vi "EJERCICIO 2 DE LOGICA COMBINACIONAL.vi"() -> ()   [LabVIEW 2013]
panel:
  out "Boolean":bool
  in  "C":bool
  in  "B":bool
  in  "A":bool
  # "universidad de cundinamarca\ningenieria de sistemas \nandy leandro camargo \nelectiva pro IV"
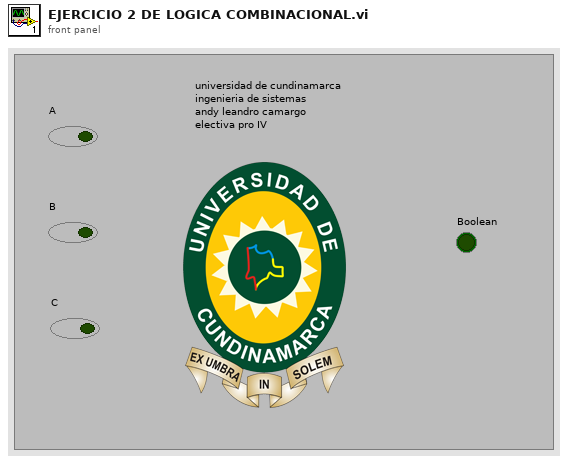
[diagram p1: front panel]
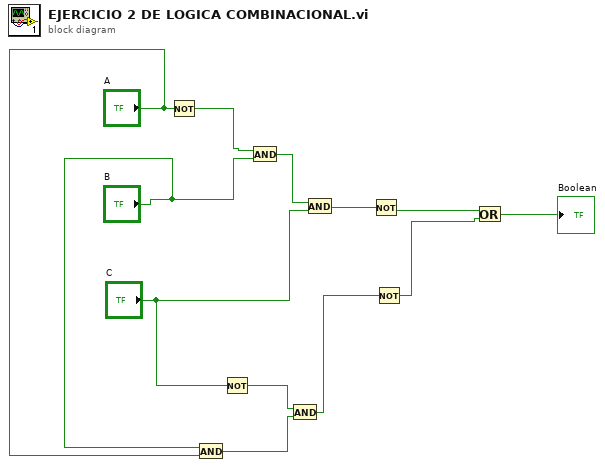
[diagram p0: block diagram]
diagram:
  n1 = Not(x="A") -> (.not. x?=w12:bool)
  n2 = And(x="B", y="A") -> (x .and. y?=w2:bool)
  n3 = Not(x="C") -> (.not. x?=w3:bool)
  n4 = And(x=w12, y="B") -> (x .and. y?=w11:bool)
  n5 = And(x=w3, y=w2) -> (x .and. y?=w1:bool)
  n6 = And(x=w11, y="C") -> (x .and. y?=w8:bool)
  n7 = Not(x=w8) -> (.not. x?=w9:bool)
  n8 = Not(x=w1) -> (.not. x?=w7:bool)
  n9 = Or(x=w9, y=w7) -> (x .or. y?=→"Boolean":bool)
